vi "host.vi"() -> ()   [LabVIEW 2020]
uses:
  <vilib>/FPGAPlugInAG/cRIO-9054/niLvFpga_Open_cRIO-9054.vi
  <vilib>/FPGAPlugInAG/cRIO-9054/niLvFpga_Reset_cRIO-9054.vi
  <vilib>/Utility/error.llb/Error Cluster From Error Code.vi
  <vilib>/rvi/errors/niLvFpgaAdjustHostInterfaceError.vi
  <vilib>/FPGAPlugInAG/cRIO-9054/niLvFpga_Run_cRIO-9054.vi
  <vilib>/FPGAPlugInAG/cRIO-9054/niLvFpga_Close_cRIO-9054.vi
  <vilib>/rvi/interface/nirviOpenFPGA/nirviOpenFPGA.xnode
  FPGA Bitfiles/sortproject_FPGATarget_FPGAbubbleSCTLFI_WSzEnHSg36Q.lvbitx
  <vilib>/rvi/interface/nirviMethod/nirviMethod.xnode
  <vilib>/rvi/interface/nirviReadWriteControl/nirviReadWriteControl.xnode
  <vilib>/rvi/interface/nirviCloseFPGA/nirviCloseFPGA.xnode
  <vilib>/Analysis/NI_AALBase.lvlib
  <vilib>/rvi/errors/niLvFpgaMergeErrorWithErrorCode.vi
  <vilib>/FPGAPlugInAG/cRIO-9054/niLvFpga_StartFifo_cRIO-9054.vi
  <vilib>/FPGAPlugInAG/cRIO-9054/niLvFpga_WriteFifo_cRIO-9054.vi
  NiFpgaLv.dll
  <vilib>/FPGAPlugInAG/cRIO-9054/niLvFpga_ReadFifo_cRIO-9054.vi
panel:
  out "sort time (ms)":dbl
  out "Elements Remaining":u32
  out "sorted signal":sgl[](graph)
  out "unsorted signal":dbl[](graph)
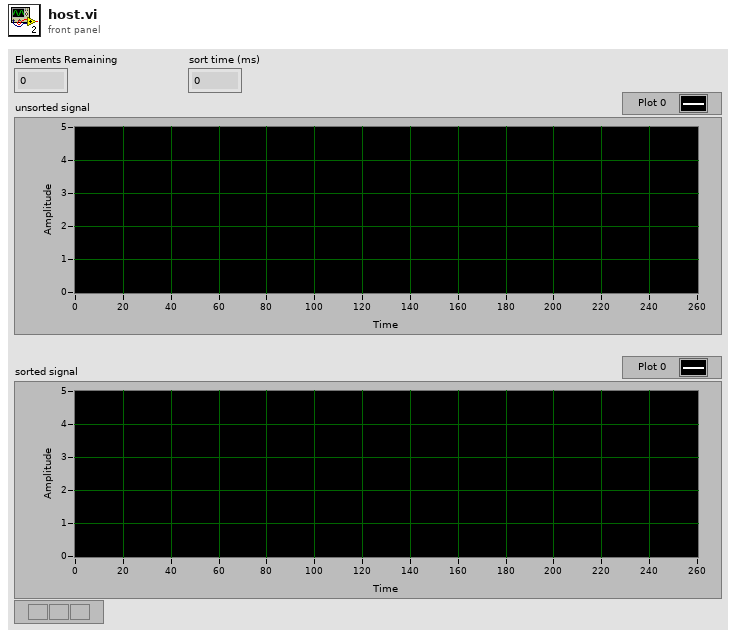
[diagram p1: front panel]
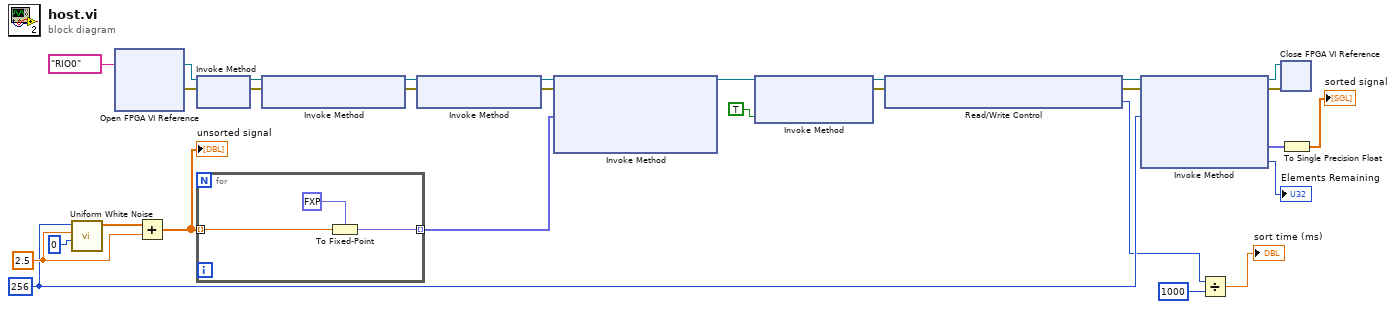
[diagram p0: block diagram]
diagram:
  w17 = 2.5 ("amplitude")
  w11 = 256
  n1 = call <vilib>:"Uniform White Noise.vi"("seed"=0, "amplitude"=w17, "samples"=w11) -> ("uniform white noise"=w18:dbl[])  [unwired: 7 in, 1 out]
  n2 = xnode "Open FPGA VI Reference"("resource name"=tag "RIO0") -> ("FPGA VI Reference Out"=w23:refnum<k20>, "error out"=w22:errorcluster)  [unwired: 1 in]
  n3 = Add(x=w18, y=w17) -> (x+y=w16:dbl[])
  "unsorted signal" <- w16
  n4 = xnode "Invoke Method"("FPGA VI Reference In"=w23, "error in"=w22) -> ("FPGA VI Reference Out"=w29:refnum<k20>, "error out"=w24:errorcluster)
  n5 = for {
    tunnel: w16 -> [w31] mode=indexing
    tunnel: [w30] -> w10 mode=indexing
    n6 = To Fixed-Point(fixed-point type=fxp<+/-,16,4> 0.0, number=w31) -> (fixed-point=w30:fxp<+/-,16,4>)
  }
  n7 = xnode "Invoke Method"("FPGA VI Reference In"=w29, "error in"=w24) -> ("FPGA VI Reference Out"=w28:refnum<k20>, "error out"=w27:errorcluster)
  n8 = xnode "Invoke Method"("FPGA VI Reference In"=w28, "error in"=w27) -> ("FPGA VI Reference Out"=w26:refnum<k20>, "error out"=w25:errorcluster)
  n9 = xnode "Invoke Method"("FPGA VI Reference In"=w26, "error in"=w25, "Data"=w10) -> ("FPGA VI Reference Out"=w8:refnum<k20>)  [unwired: 1 in, 2 out]
  n10 = xnode "Invoke Method"("FPGA VI Reference In"=w8, "Wait Until Done (F)"=TRUE) -> ("FPGA VI Reference Out"=w7:refnum<k20>, "error out"=w6:errorcluster)  [unwired: 1 in]
  n11 = xnode "Read/Write Control"("FPGA VI Reference In"=w7, "error in"=w6) -> ("FPGA VI Reference Out"=w5:refnum<k20>, "error out"=w4:errorcluster, "sort time (us)"=w3:u32)
  n12 = xnode "Invoke Method"("FPGA VI Reference In"=w5, "error in"=w4, "Number of Elements"=w11) -> ("FPGA VI Reference Out"=w20:refnum<k20>, "error out"=w21:errorcluster, "Data"=w15:fxp<+/-,16,4>[], "Elements Remaining"=→"Elements Remaining":u32)  [unwired: 1 in]
  n13 = Divide(x=w3, y=u32 1000) -> (x/y=→"sort time (ms)":dbl)
  n14 = xnode "Close FPGA VI Reference"("FPGA VI Reference In"=w20, "error in"=w21) -> ()  [unwired: 1 out]
  n15 = To Single Precision Float(number=w15) -> (single precision float=→"sorted signal":sgl[])
